vi "Chirp_OOP.vi"() -> ()   [LabVIEW 2014, in "ChirpEIS.lvclass"]
uses:
  ChirpEIS.lvclass
  States.ctl
  ChirpEIS.lvclass/ChirpEIS.ctl
panel:
  in  "Chirp control":T1={"R external(Ohm)"=96.0, "Chirp Start(Hz)"=0.1, "Chirp Ends(Hz)"=10.0, "Vmin"=0.0, "VInc"=0.2, "Vmax"=0.8, "Chirp T(s)"=0.8}
  out "error out":errorcluster
  out "data 2":dynamicdata(graph) caption="data"
  out "DC bias":dbl
  out "State":T2=enum."IncreaseVoltage"
  in  "stop":bool
  in  "Setup":string="R = 150 C = 1000uF Rleak = 1000Ohm"
  in  "Path":path=path "C:/Users/YuanYuan/Desktop/Labview Data/Chirp"
  in  "ChirpEIS.lvclass":refnum<class "ChirpEIS.lvclass">
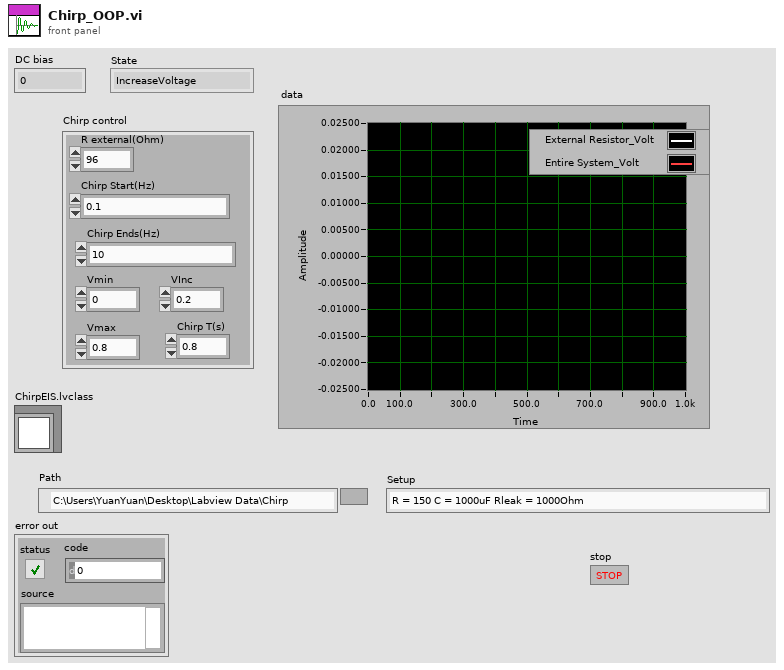
[diagram p1: front panel]
types:
  T1 = cluster{"R external(Ohm)":dbl, "Chirp Start(Hz)":dbl, "Chirp Ends(Hz)":dbl, "Vmin":dbl, "VInc":dbl, "Vmax":dbl, "Chirp T(s)":dbl}
  T2 = typedef "States.ctl" = enum16{"AddDuration", "AddFreq", "CreateNewFile", "Wait", "IncreaseVoltage", "DFT", "ChirpMeasurement", "Initialize", "Ternimate"}
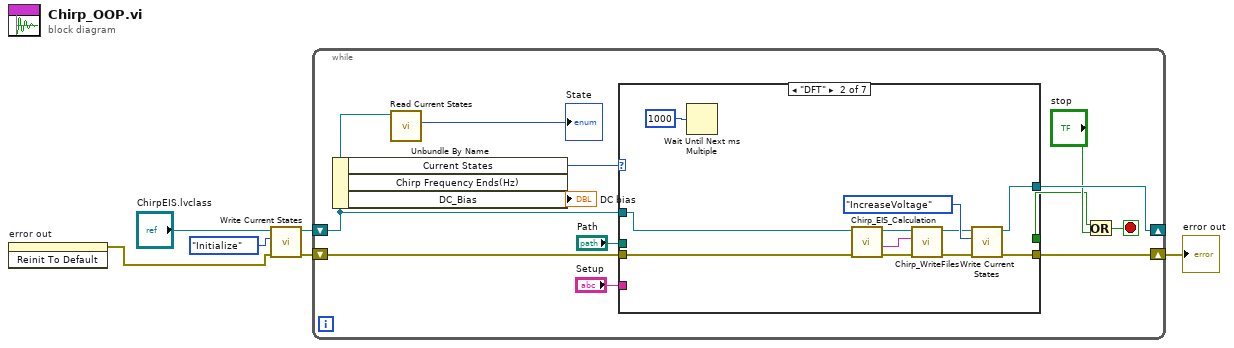
[diagram p0: block diagram]
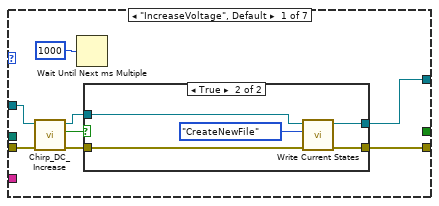
[diagram p2: hidden frame]
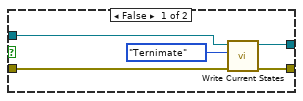
[diagram p3: hidden frame]
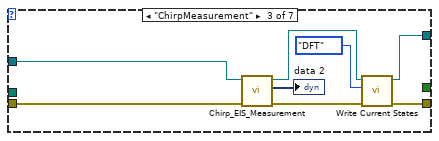
[diagram p4: hidden frame]
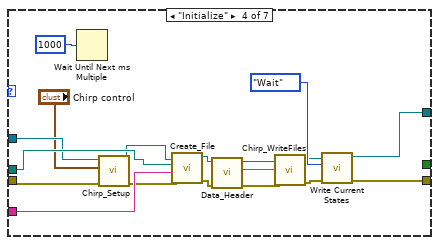
[diagram p5: hidden frame]
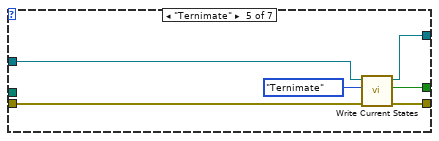
[diagram p6: hidden frame]
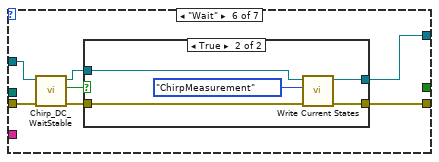
[diagram p7: hidden frame]
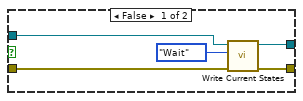
[diagram p8: hidden frame]
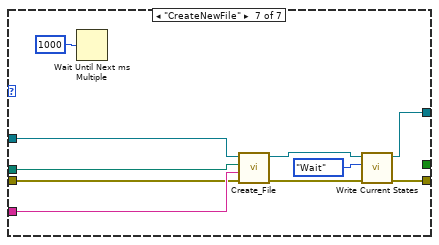
[diagram p9: hidden frame]
diagram:
  n1 = invoke on="error out" class="Clust (strict)" method="Reinit To Default"() -> (error out=w1:errorcluster)  [unwired: 3 in, 2 out]
  n2 = call-dynamic "Write Current States.vi"("error in (no error)"=w1, "Enum"=States."Initialize", "ChirpEIS in"="ChirpEIS.lvclass") -> ("error out"=w3:errorcluster, "ChirpEIS out"=w5:refnum<class "ChirpEIS.lvclass">)  [unwired: 6 in, 1 out]
  n3 = while {
    shift-right: [w16] -> _
    shift-left: w5 -> [w14]
    shift-right: [w15] -> w2
    shift-left: w3 -> [w17]
    stop <- w10 stop-if-true
    n4 = Unbundle By Name(w14) -> ("Current States"=w18:T2, "DC_Bias"=→"DC bias":dbl)  [unwired: 1 out]
    n5 = call-dynamic "Read Current States.vi"("ChirpEIS in"=w14) -> ("Enum"=→"State":T2)  [unwired: 8 in, 2 out]
    n6 = case shown="\"DFT\"" w18 {
      tunnel: w14 -> [w23 w44 w48 w62 w79 w83 w104]
      tunnel: w17 -> [w20 w43 w52 w61 w78 w82 w103]
      tunnel: [w26 w46 w54 w72 w77 w86 w102] -> w16
      tunnel: [w25 w45 w53 w71 w76 w85 w101] -> w15
      tunnel: [_ _ _ _ w74 _ _] -> w11
      tunnel: "Path" -> [_ _ _ w70 _ _ w106]
      tunnel: "Setup" -> [_ _ _ w69 _ _ w105]
      frame "IncreaseVoltage", Default {
        n7 = call-dynamic "Chirp_DC_Increase.vi"("error in (no error)"=w20, "ChirpEIS in"=w23) -> ("error out"=w21:errorcluster, "Less than Max DC"=w24:bool, "ChirpEIS out"=w22:refnum<class "ChirpEIS.lvclass">)  [unwired: 7 in]
        n8 = Wait Until Next ms Multiple(millisecond multiple=u32 1000) -> ()  [unwired: 1 out]
        n9 = case shown="True" w24 {
          tunnel: w22 -> [w28 w36]
          tunnel: w21 -> [w27 w35]
          tunnel: [w30 w34] -> w26
          tunnel: [w29 w33] -> w25
          frame False {
            n10 = call-dynamic "Write Current States.vi"("error in (no error)"=w27, "Enum"=States."Ternimate", "ChirpEIS in"=w28) -> ("error out"=w29:errorcluster, "ChirpEIS out"=w30:refnum<class "ChirpEIS.lvclass">)  [unwired: 6 in, 1 out]
          }
          frame True {
            n11 = call-dynamic "Write Current States.vi"("error in (no error)"=w35, "Enum"=States."CreateNewFile", "ChirpEIS in"=w36) -> ("error out"=w33:errorcluster, "ChirpEIS out"=w34:refnum<class "ChirpEIS.lvclass">)  [unwired: 6 in, 1 out]
          }
        }
      }
      frame "DFT" {
        n12 = Wait Until Next ms Multiple(millisecond multiple=u32 1000) -> ()  [unwired: 1 out]
        n13 = call-dynamic "Chirp_EIS_Calculation.vi"("error in (no error)"=w43, "ChirpEIS in"=w44) -> ("error out"=w40:errorcluster, "EIS Results"=w42:string, "ChirpEIS out"=w41:refnum<class "ChirpEIS.lvclass">)  [unwired: 6 in, 1 out]
        n14 = call-dynamic "Chirp_WriteFiles.vi"("error in (no error)"=w40, "Data"=w42, "ChirpEIS in"=w41) -> ("error out"=w38:errorcluster, "ChirpEIS out"=w39:refnum<class "ChirpEIS.lvclass">)  [unwired: 7 in]
        n15 = call-dynamic "Write Current States.vi"("error in (no error)"=w38, "Enum"=States."IncreaseVoltage", "ChirpEIS in"=w39) -> ("error out"=w45:errorcluster, "ChirpEIS out"=w46:refnum<class "ChirpEIS.lvclass">)  [unwired: 6 in, 1 out]
      }
      frame "ChirpMeasurement" {
        n16 = call-dynamic "Chirp_EIS_Measurement.vi"("error in (no error)"=w52, "ChirpEIS in"=w48) -> ("error out"=w50:errorcluster, "data"=→"data 2":dynamicdata, "ChirpEIS out"=w51:refnum<class "ChirpEIS.lvclass">)  [unwired: 5 in, 2 out]
        n17 = call-dynamic "Write Current States.vi"("error in (no error)"=w50, "Enum"=States."DFT", "ChirpEIS in"=w51) -> ("error out"=w53:errorcluster, "ChirpEIS out"=w54:refnum<class "ChirpEIS.lvclass">)  [unwired: 6 in, 1 out]
      }
      frame "Initialize" {
        n18 = Wait Until Next ms Multiple(millisecond multiple=u32 1000) -> ()  [unwired: 1 out]
        n19 = call "Chirp_Setup.vi"("error in (no error)"=w61, "Chirp control"="Chirp control", "ChirpEIS in"=w62) -> ("error out"=w59:errorcluster, "ChirpEIS out"=w60:refnum<class "ChirpEIS.lvclass">)  [unwired: 7 in]
        n20 = call "Create_File.vi"("error in (no error)"=w59, "Setup"=w69, "Path"=w70, "ChirpEIS in"=w60) -> ("error out"=w57:errorcluster, "ChirpEIS out"=w58:refnum<class "ChirpEIS.lvclass">)  [unwired: 6 in]
        n21 = call-dynamic "Data_Header.vi"("error in (no error)"=w57, "ChirpEIS in"=w58) -> ("error out"=w63:errorcluster, "Header String"=w64:string, "ChirpEIS out"=w65:refnum<class "ChirpEIS.lvclass">)  [unwired: 7 in]
        n22 = call-dynamic "Chirp_WriteFiles.vi"("error in (no error)"=w63, "Data"=w64, "ChirpEIS in"=w65) -> ("error out"=w66:errorcluster, "ChirpEIS out"=w67:refnum<class "ChirpEIS.lvclass">)  [unwired: 7 in]
        n23 = call-dynamic "Write Current States.vi"("error in (no error)"=w66, "Enum"=States."Wait", "ChirpEIS in"=w67) -> ("error out"=w71:errorcluster, "ChirpEIS out"=w72:refnum<class "ChirpEIS.lvclass">)  [unwired: 6 in, 1 out]
      }
      frame "Ternimate" {
        n24 = call-dynamic "Write Current States.vi"("error in (no error)"=w78, "Enum"=States."Ternimate", "ChirpEIS in"=w79) -> ("error out"=w76:errorcluster, "Boolean"=w74:bool, "ChirpEIS out"=w77:refnum<class "ChirpEIS.lvclass">)  [unwired: 6 in]
      }
      frame "Wait" {
        n25 = call-dynamic "Chirp_DC_WaitStable.vi"("error in (no error)"=w82, "ChirpEIS in"=w83) -> ("error out"=w80:errorcluster, "logical AND"=w84:bool, "ChirpEIS out"=w81:refnum<class "ChirpEIS.lvclass">)  [unwired: 6 in, 1 out]
        n26 = case shown="True" w84 {
          tunnel: w81 -> [w88 w96]
          tunnel: w80 -> [w87 w95]
          tunnel: [w90 w94] -> w86
          tunnel: [w89 w93] -> w85
          frame False {
            n27 = call-dynamic "Write Current States.vi"("error in (no error)"=w87, "Enum"=States."Wait", "ChirpEIS in"=w88) -> ("error out"=w89:errorcluster, "ChirpEIS out"=w90:refnum<class "ChirpEIS.lvclass">)  [unwired: 6 in, 1 out]
          }
          frame True {
            n28 = call-dynamic "Write Current States.vi"("error in (no error)"=w95, "Enum"=States."ChirpMeasurement", "ChirpEIS in"=w96) -> ("error out"=w93:errorcluster, "ChirpEIS out"=w94:refnum<class "ChirpEIS.lvclass">)  [unwired: 6 in, 1 out]
          }
        }
      }
      frame "CreateNewFile" {
        n29 = Wait Until Next ms Multiple(millisecond multiple=u32 1000) -> ()  [unwired: 1 out]
        n30 = call "Create_File.vi"("error in (no error)"=w103, "Setup"=w105, "Path"=w106, "ChirpEIS in"=w104) -> ("error out"=w99:errorcluster, "ChirpEIS out"=w100:refnum<class "ChirpEIS.lvclass">)  [unwired: 6 in]
        n31 = call-dynamic "Write Current States.vi"("error in (no error)"=w99, "Enum"=States."Wait", "ChirpEIS in"=w100) -> ("error out"=w101:errorcluster, "ChirpEIS out"=w102:refnum<class "ChirpEIS.lvclass">)  [unwired: 6 in, 1 out]
      }
    }
    n32 = Or(x=w11, y="stop") -> (x .or. y?=w10:bool)
  }
  "error out" <- w2
